vi "latch.vi"(10 "in":dbl, 11 "condition":bool) -> (3 "latch out":dbl)   [LabVIEW 2014]
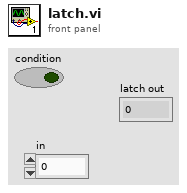
[diagram p1: front panel]
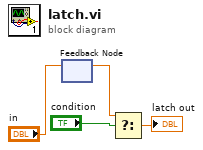
[diagram p0: block diagram]
diagram:
  n1 = feedback #1() -> (w2:dbl)  [unwired: 1 in]
  n2 = feedback-in #1("in") -> ()
  n3 = Select(t=w2, s="condition") -> (s? t:f=→"latch out":dbl)  [unwired: 1 in]
